vi "Do.vi"(8 "error in (no error)":errorcluster, 10 "FormulaG API":refnum<class "FormulaG API.lvclass">, 11 "Select Cam Cmd in":refnum<class "Select Cam Cmd.lvclass">) -> (0 "error out":errorcluster, 3 "Select Cam Cmd out":refnum<class "Select Cam Cmd.lvclass">)   [LabVIEW 2024, in "FormulaG.lvlib" / "Select Cam Cmd.lvclass"]
uses:
  Select Cam Cmd.lvclass
  FormulaG API/FormulaG API.lvclass
  Select Cam Cmd.lvclass/Select Cam Cmd.ctl
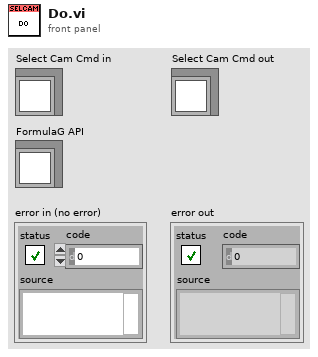
[diagram p1: front panel]
types:
  T1 = typedef "FormulaG-Common.lvlib/Camera.ctl" = enum16{"Chase", "Overhead"}
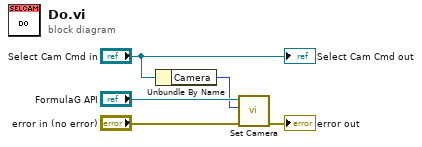
[diagram p0: block diagram]
diagram:
  n1 = Unbundle By Name("Select Cam Cmd in") -> ("Camera"=w1:T1)
  n2 = call "Set Camera.vi"("error in (no error)"="error in (no error)", "Camera"=w1, "FormulaG API in"="FormulaG API") -> ("error out"=→"error out":errorcluster)  [unwired: 7 in, 1 out]
  "Select Cam Cmd out" <- "Select Cam Cmd in"
